vi "Initialize Datasheets List.vi"(8 "error in (no error)":errorcluster, 9 "Test Type (List at Top)":string, 10 "Selected Datasheet Keys (none)":i32[](array[numeric]), 11 "Datasheets Control":refnum<vi>) -> (0 "error out":errorcluster, 1 "Disabled Items":i32[](array[numeric]), 2 "Selected Datasheets":i32[](array[numeric]), 3 "Available Datasheets":string[](array[string]))   [LabVIEW 2011]
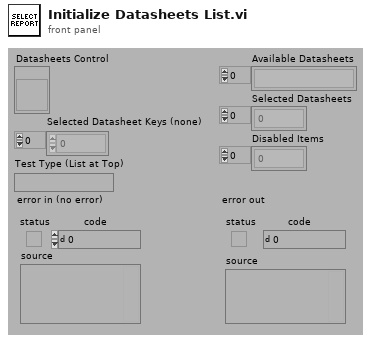
[diagram p1: front panel]
types:
  T1 = typedef "Template Record.ctl" = cluster{"Title":string, "KEY":i32, "Path":path, "Description":string, "Type":string, "Processing":string, "Parameters":string}
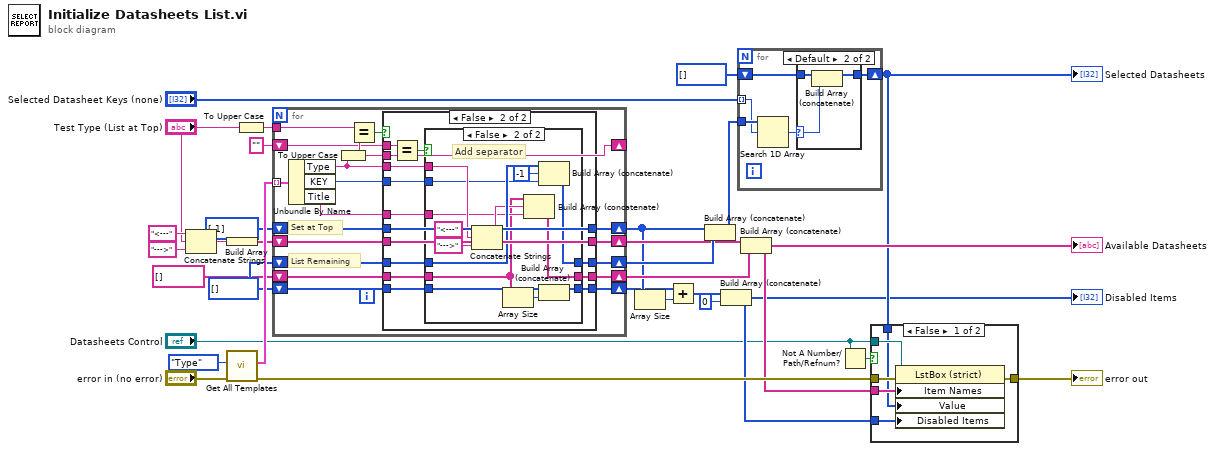
[diagram p0: block diagram]
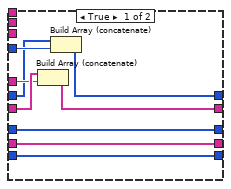
[diagram p4: hidden frame]
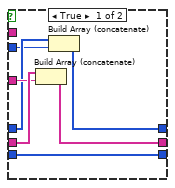
[diagram p5: hidden frame]
diagram:
  w9 = i32[] [] ("Selected Reports")
  n1 = Concatenate Strings("<---" ("string"), "Test Type (List at Top)", "--->" ("string")) -> (w4:string)
  n2 = Build Array(w4) -> (w5:string[])
  n3 = call "Get All Templates.vi"("error in (no error)"="error in (no error)", "Order By (Title)"=enum16{"Title", "Type"}."Type") -> ("error out"=w21:errorcluster, "Templates"=w30:T1[])  [unwired: 2 in, 6 out]
  n4 = To Upper Case(1:"Test Type (List at Top)") -> (0:w23:string)
  n5 = for {
    tunnel: w30 -> [w49] mode=indexing
    tunnel: w23 -> [w48]
    shift-right: [w39] -> w13
    shift-left: i32[] [-1] ("Selected Reports") -> [w44]
    shift-right: [w40] -> w25
    shift-left: w5 -> [w43]
    shift-right: [w37] -> w26
    shift-left: w9 -> [w42]
    shift-right: [w38] -> w24
    shift-left: string[] [] -> [w41]
    shift-right: [w36] -> _
    shift-left: "" ("Type") -> [w35]
    shift-right: [w32] -> w11
    shift-left: w9 -> [w33]
    # "List Remaining"
    # "Set at Top"
    n6 = Unbundle By Name(w49) -> ("Type"=w34:string, "KEY"=w46:i32, "Title"=w45:string)
    n7 = To Upper Case(1:w34) -> (0:w36:string)
    n8 = Equal?(x=w48, y=w36) -> (x = y?=w47:bool)
    n9 = case shown="False" w47 {
      tunnel: w46 -> [w53 w72]
      tunnel: w45 -> [w54 w71]
      tunnel: w44 -> [w50 w66]
      tunnel: w43 -> [w58 w65]
      tunnel: w42 -> [w57 w69]
      tunnel: w41 -> [w56 w70]
      tunnel: [w51 w65] -> w40
      tunnel: [w52 w66] -> w39
      tunnel: [w56 w68] -> w38
      tunnel: [w57 w67] -> w37
      tunnel: w36 -> [_ w64]
      tunnel: w35 -> [_ w63]
      tunnel: w34 -> [_ w61]
      tunnel: w33 -> [w55 w60]
      tunnel: [w55 w59] -> w32
      frame True {
        n10 = Build Array (concatenate)(w58, w54) -> (w51:string[])
        n11 = Build Array (concatenate)(w50, w53) -> (w52:i32[])
      }
      frame False {
        n12 = Equal?(x=w63, y=w64) -> (x = y?=w62:bool)
        n13 = case shown="False" w62 {
          tunnel: w72 -> [w75 w83]
          tunnel: w71 -> [w77 w85]
          tunnel: w70 -> [w79 w81]
          tunnel: w69 -> [w76 w93]
          tunnel: [w73 w84] -> w68
          tunnel: [w74 w82] -> w67
          tunnel: w61 -> [_ w88]
          tunnel: w60 -> [w78 w87]
          tunnel: [w78 w86] -> w59
          frame True {
            n14 = Build Array (concatenate)(w79, w77) -> (w73:string[])
            n15 = Build Array (concatenate)(w76, w75) -> (w74:i32[])
          }
          frame False {
            # "Add separator"
            n16 = Concatenate Strings("<---" ("string"), w88, "--->" ("string")) -> (w89:string)
            n17 = Array Size(array=w81) -> (size(s)=w80:i32)
            n18 = Build Array (concatenate)(w81, w89, w85) -> (w84:string[])
            n19 = Build Array (concatenate)(w93, -1 ("element"), w83) -> (w82:i32[])
            n20 = Build Array (concatenate)(w87, w80) -> (w86:i32[])
          }
        }
      }
    }
  }
  n21 = Array Size(array=w13) -> (size(s)=w12:i32)
  n22 = Add(x=w11, y=w12) -> (x+y=w3:i32[])
  n23 = Build Array (concatenate)(w13, w26) -> (w18:i32[])
  n24 = Build Array (concatenate)(w3, 0 ("Numeric")) -> (w8:i32[])
  "Disabled Items" <- w8
  n25 = for {
    shift-right: [w95] -> w17
    shift-left: i32[] [] ("Selected Reports") -> [w96]
    tunnel: w18 -> [w98]
    tunnel: "Selected Datasheet Keys (none)" -> [w94] mode=indexing
    n26 = Search 1D Array(1D array=w98, element=w94) -> (index of element=w97:i32)  [unwired: 1 out]
    n27 = case shown="Default" w97 {
      selector: w97 -> [_ w100]
      tunnel: [w99 w101] -> w95
      tunnel: w96 -> [w99 w102]
      frame -1 {
      }
      frame Default {
        n28 = Build Array (concatenate)(w102, w100) -> (w101:i32[])
      }
    }
  }
  "Selected Datasheets" <- w17
  n29 = Build Array (concatenate)(w25, w24) -> (w19:string[])
  "Available Datasheets" <- w19
  n30 = Not A Number/Path/Refnum?(number/path/refnum="Datasheets Control") -> (NaN/Path/Refnum?=w1:bool)
  n31 = case shown="False" w1 {
    tunnel: w21 -> [w108 w109]
    tunnel: [w107 w109] -> w20
    tunnel: "Datasheets Control" -> [w106 _]
    tunnel: w19 -> [w105 _]
    tunnel: w17 -> [w104 _]
    tunnel: w8 -> [w103 _]
    frame False {
      n32 = property class="LstBox (strict)"(reference=w106, error in=w108, "Item Names"=w105, "Value"=w104, "Disabled Items"=w103) -> (error out=w107:errorcluster)  [unwired: 1 out]
    }
    frame True {
    }
  }
  "error out" <- w20
